vi "Rtde.vi"() -> ()   [LabVIEW 2019]
uses:
  C:/Users/fg/Documents/UniversalRobots.vi/LabVIEW_2024/UnderAutomation.UniversalRobots/lib/UnderAutomation.UniversalRobots.dll
  LabVIEW_2024/UnderAutomation.UniversalRobots/lib/UnderAutomation.UniversalRobots.dll
panel:
  out "Int11":i32
  out "StandardAnalogInput0":dbl
  out "Waveform Z":dbl(graph)
  in  "stop":bool
  in  "Speed":dbl(slide) scale=0.0..1.0
  out "Connected":bool
  out "Error logs":string
  out "Connect error":errorcluster
  # "RTDE with LabVIEW"
  # "Use stop button to properly stop RTDE"
  # "SEND INPUT VALUES"
  # "OUTPUT VALUES EXAMPLE : TCP X at 500HZ"
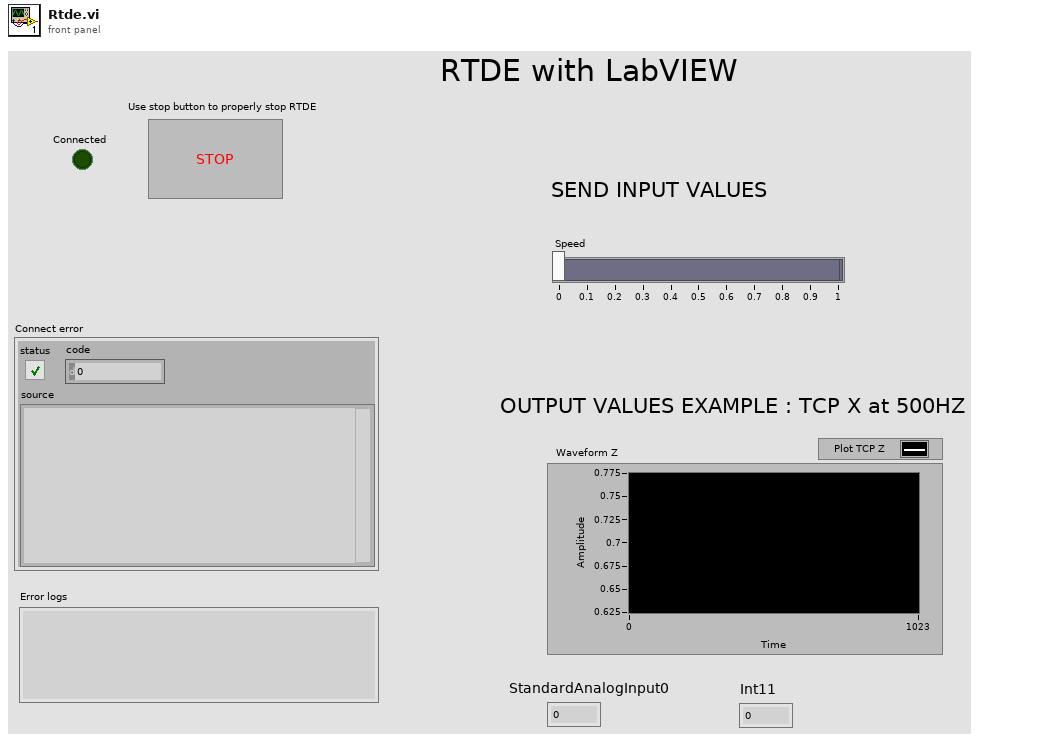
[diagram p1: front panel]
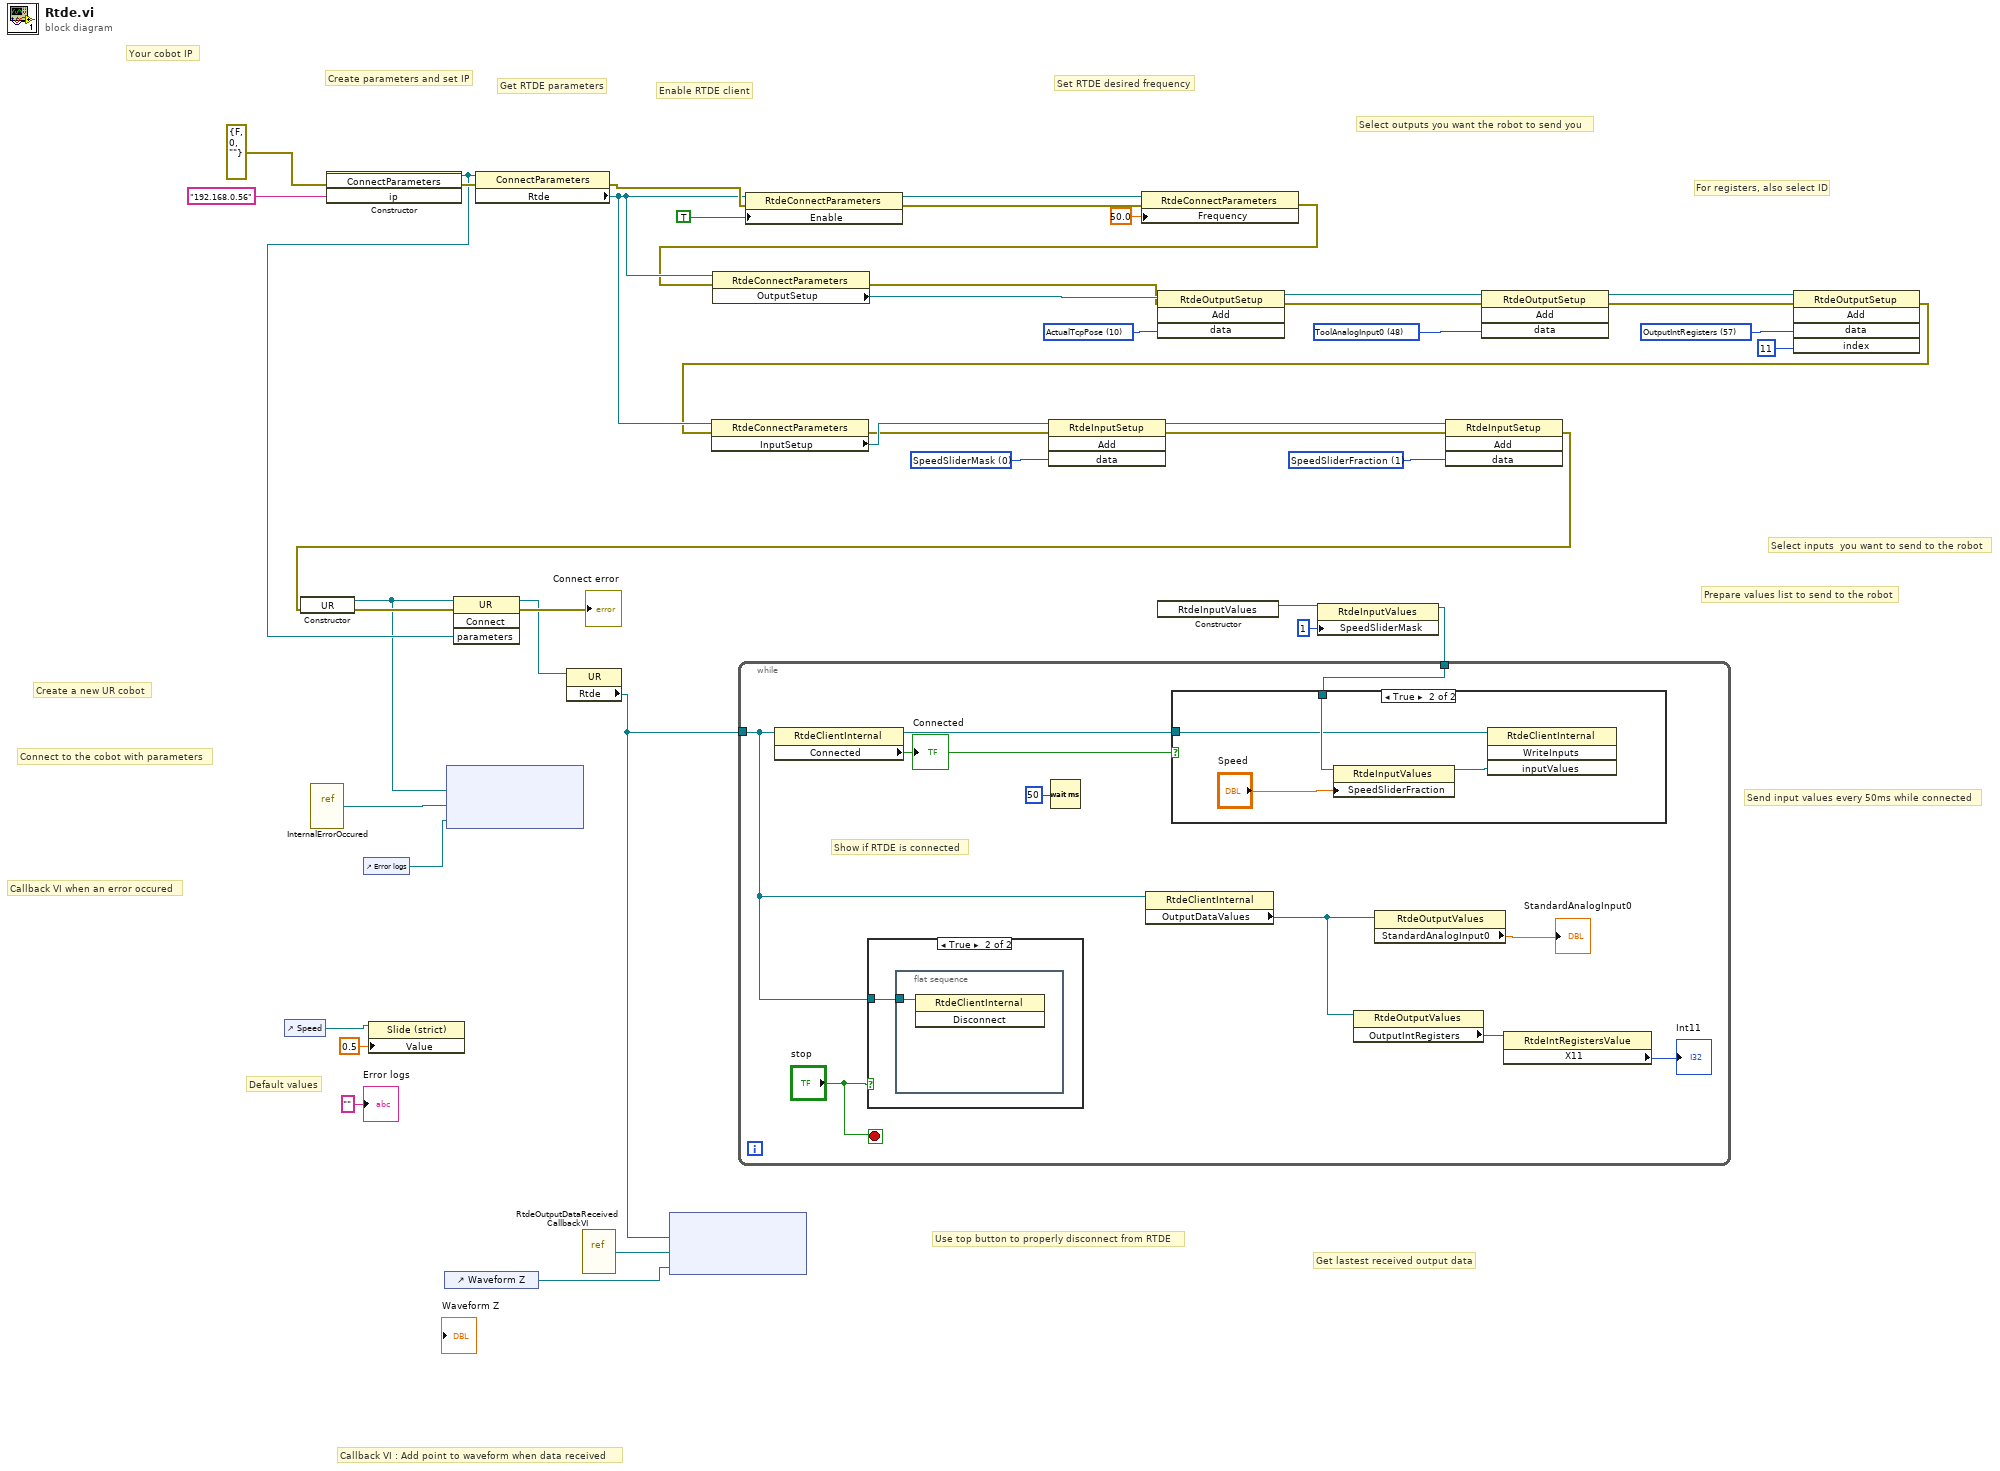
[diagram p0: block diagram]
diagram:
  w26 = 1 items=["SpeedSliderMask", "SpeedSliderFraction", "StandardDigitalOutputMask", "ConfigurableDigitalOutputMask", "StandardDigitalOutput", "ConfigurableDigitalOutput", "StandardAnalogOutputMask", "StandardAnalogOutputType", "StandardAnalogOutput0", "StandardAnalogOutput1", "InputBtRegisters0To31", "InputBtRegisters32To63", "InputBitRegisters", "InputIntRegisters", "InputDoubleRegisters", "ExternalForceTorque"] ("data")
  w28 = 0 items=["SpeedSliderMask", "SpeedSliderFraction", "StandardDigitalOutputMask", "ConfigurableDigitalOutputMask", "StandardDigitalOutput", "ConfigurableDigitalOutput", "StandardAnalogOutputMask", "StandardAnalogOutputType", "StandardAnalogOutput0", "StandardAnalogOutput1", "InputBtRegisters0To31", "InputBtRegisters32To63", "InputBitRegisters", "InputIntRegisters", "InputDoubleRegisters", "ExternalForceTorque"] ("data")
  w38 = 57 items=["Timestamp", "TargetQ", "TargetQd", "TargetQdd", "TargetCurrent", "TargetMoment", "ActualQ", "ActualQd", "ActualCurrent", "JointControlOutput", "ActualTcpPose", "ActualTcpSpeed", "ActualTcpForce", "TargetTcpPose", "TargetTcpSpeed", "ActualDigitalInputBits", "JointTemperatures", "ActualExecutionTime", "RobotMode", "JointMode", "SafetyMode", "SafetyStatus", "ActualToolAccelerometer", "SpeedScaling", "TargetSpeedFraction", "ActualMomentum", "ActualMainVoltage", "ActualRobotVoltage", "ActualRobotCurrent", "ActualJointVoltage", "ActualDigitalOutputBits", "RuntimeState", "ElbowPosition", "ElbowVelocity", "RobotStatusBits", "SafetyStatusBits", "AnalogIOTypes", "StandardAnalogInput0", "StandardAnalogInput1", "StandardAnalogOutput0", "StandardAnalogOutput1", "IOCurrent", "Euromap67InputBits", "Euromap67OutputBits", "Euromap67_24VVoltage", "Euromap67_24VCurrent", "ToolMode", "ToolAnalogInputTypes", "ToolAnalogInput0", "ToolAnalogInput1", "ToolOutputVoltage", "ToolOutputCurrent", "ToolTemperature", "TcpForceScalar", "OutputBitRegisters0To31", "OutputBitRegisters32To63", "OutputBitRegisters", "OutputIntRegisters", "OutputDoubleRegisters", "InputBitRegisters0To31", "InputBitRegisters32To63", "InputBitRegisters", "InputIntRegisters", "InputDoubleRegisters", "ToolOutputMode", "ToolDigitalOutput0mode", "ToolDigitalOutput1Mode", "Payload", "PayloadCOG", "PayloadInertia", "ScriptControlLine", "FTRawWrench"] ("data")
  w40 = 48 items=["Timestamp", "TargetQ", "TargetQd", "TargetQdd", "TargetCurrent", "TargetMoment", "ActualQ", "ActualQd", "ActualCurrent", "JointControlOutput", "ActualTcpPose", "ActualTcpSpeed", "ActualTcpForce", "TargetTcpPose", "TargetTcpSpeed", "ActualDigitalInputBits", "JointTemperatures", "ActualExecutionTime", "RobotMode", "JointMode", "SafetyMode", "SafetyStatus", "ActualToolAccelerometer", "SpeedScaling", "TargetSpeedFraction", "ActualMomentum", "ActualMainVoltage", "ActualRobotVoltage", "ActualRobotCurrent", "ActualJointVoltage", "ActualDigitalOutputBits", "RuntimeState", "ElbowPosition", "ElbowVelocity", "RobotStatusBits", "SafetyStatusBits", "AnalogIOTypes", "StandardAnalogInput0", "StandardAnalogInput1", "StandardAnalogOutput0", "StandardAnalogOutput1", "IOCurrent", "Euromap67InputBits", "Euromap67OutputBits", "Euromap67_24VVoltage", "Euromap67_24VCurrent", "ToolMode", "ToolAnalogInputTypes", "ToolAnalogInput0", "ToolAnalogInput1", "ToolOutputVoltage", "ToolOutputCurrent", "ToolTemperature", "TcpForceScalar", "OutputBitRegisters0To31", "OutputBitRegisters32To63", "OutputBitRegisters", "OutputIntRegisters", "OutputDoubleRegisters", "InputBitRegisters0To31", "InputBitRegisters32To63", "InputBitRegisters", "InputIntRegisters", "InputDoubleRegisters", "ToolOutputMode", "ToolDigitalOutput0mode", "ToolDigitalOutput1Mode", "Payload", "PayloadCOG", "PayloadInertia", "ScriptControlLine", "FTRawWrench"] ("data")
  w42 = 10 items=["Timestamp", "TargetQ", "TargetQd", "TargetQdd", "TargetCurrent", "TargetMoment", "ActualQ", "ActualQd", "ActualCurrent", "JointControlOutput", "ActualTcpPose", "ActualTcpSpeed", "ActualTcpForce", "TargetTcpPose", "TargetTcpSpeed", "ActualDigitalInputBits", "JointTemperatures", "ActualExecutionTime", "RobotMode", "JointMode", "SafetyMode", "SafetyStatus", "ActualToolAccelerometer", "SpeedScaling", "TargetSpeedFraction", "ActualMomentum", "ActualMainVoltage", "ActualRobotVoltage", "ActualRobotCurrent", "ActualJointVoltage", "ActualDigitalOutputBits", "RuntimeState", "ElbowPosition", "ElbowVelocity", "RobotStatusBits", "SafetyStatusBits", "AnalogIOTypes", "StandardAnalogInput0", "StandardAnalogInput1", "StandardAnalogOutput0", "StandardAnalogOutput1", "IOCurrent", "Euromap67InputBits", "Euromap67OutputBits", "Euromap67_24VVoltage", "Euromap67_24VCurrent", "ToolMode", "ToolAnalogInputTypes", "ToolAnalogInput0", "ToolAnalogInput1", "ToolOutputVoltage", "ToolOutputCurrent", "ToolTemperature", "TcpForceScalar", "OutputBitRegisters0To31", "OutputBitRegisters32To63", "OutputBitRegisters", "OutputIntRegisters", "OutputDoubleRegisters", "InputBitRegisters0To31", "InputBitRegisters32To63", "InputBitRegisters", "InputIntRegisters", "InputDoubleRegisters", "ToolOutputMode", "ToolDigitalOutput0mode", "ToolDigitalOutput1Mode", "Payload", "PayloadCOG", "PayloadInertia", "ScriptControlLine", "FTRawWrench"] ("data")
  # "Use top button to properly disconnect from RTDE"
  # "Get lastest received output data"
  # "Send input values every 50ms while connected"
  # "Prepare values list to send to the robot"
  # "Callback VI : Add point to waveform when data received"
  # "Default values"
  # "Callback VI when an error occured"
  # "Connect to the cobot with parameters"
  # "Create a new UR cobot"
  # "Your cobot IP"
  # "Create parameters and set IP"
  # "Get RTDE parameters"
  # "Enable RTDE client"
  # "Set RTDE desired frequency"
  # "Select inputs  you want to send to the robot"
  # "For registers, also select ID"
  # "Select outputs you want the robot to send you"
  n1 = control-ref of="Speed"() -> (w2:refnum<vi>)
  n2 = vi-ref "InternalErrorOccured.vi"() -> ("vi reference"=w11:refnum<vi>)
  n3 = constructor class="ConnectParameters"(error in=errorcluster {"status"=FALSE, "code"=0, "source"=""} ("error in (no error)"), "ip"="192.168.0.56") -> (reference out=w16:refnum<k24>, error out=w35:errorcluster)  [unwired: 2 in, 2 out]
  n4 = control-ref of="Error logs"() -> (w12:refnum<vi>)
  n5 = property class="Slide (strict)"(reference=w2, "Value"=0.5) -> ()  [unwired: 1 in, 2 out]
  n6 = control-ref of="Waveform Z"() -> (w4:refnum<vi>)
  n7 = property class="ConnectParameters"(reference=w16, error in=w35) -> (error out=w34:errorcluster, "Rtde"=w30:refnum<k24>)  [unwired: 1 out]
  n8 = vi-ref "RtdeOutputDataReceivedCallbackVI.vi"() -> ("vi reference"=w3:refnum<vi>)
  n9 = property class="RtdeConnectParameters"(reference=w30, error in=w34, "Enable"=TRUE) -> (reference out=w22:refnum<k24>, error out=w20:errorcluster)
  n10 = property class="RtdeConnectParameters"(reference=w22, error in=w20, "Frequency"=50.0) -> (error out=w19:errorcluster)  [unwired: 1 out]
  n11 = property class="RtdeConnectParameters"(reference=w30, error in=w19) -> (error out=w33:errorcluster, "OutputSetup"=w43:refnum<k24>)  [unwired: 1 out]
  n12 = invoke class="RtdeOutputSetup" method="Add"(reference=w43, error in=w33, "data"=w42) -> (reference out=w41:refnum<k24>, error out=w32:errorcluster)  [unwired: 1 in, 2 out]
  n13 = constructor class="RtdeInputValues"() -> (reference out=w9:refnum<k24>)  [unwired: 3 in, 2 out]
  n14 = property class="RtdeInputValues"(reference=w9, "SpeedSliderMask"=u32 1) -> (reference out=w7:refnum<k24>)  [unwired: 1 in, 1 out]
  n15 = invoke class="RtdeOutputSetup" method="Add"(reference=w41, error in=w32, "data"=w40) -> (reference out=w39:refnum<k24>, error out=w31:errorcluster)  [unwired: 1 in, 2 out]
  n16 = invoke class="RtdeOutputSetup" method="Add"(reference=w39, error in=w31, "data"=w38, "index"=11) -> (error out=w25:errorcluster)  [unwired: 1 in, 4 out]
  n17 = property class="RtdeConnectParameters"(reference=w30, error in=w25) -> (error out=w24:errorcluster, "InputSetup"=w29:refnum<k24>)  [unwired: 1 out]
  n18 = invoke class="RtdeInputSetup" method="Add"(reference=w29, error in=w24, "data"=w28) -> (reference out=w27:refnum<k24>, error out=w23:errorcluster)  [unwired: 1 in, 2 out]
  n19 = invoke class="RtdeInputSetup" method="Add"(reference=w27, error in=w23, "data"=w26) -> (error out=w17:errorcluster)  [unwired: 1 in, 3 out]
  n20 = constructor class="UR"(error in=w17) -> (reference out=w6:refnum<k24>, error out=w18:errorcluster)  [unwired: 2 in, 1 out]
  n21 = node(w6, w11, w12) -> ()  [unwired: 2 in, 2 out]
  n22 = invoke class="UR" method="Connect"(reference=w6, error in=w18, "parameters"=w16) -> (reference out=w13:refnum<k24>, error out=→"Connect error":errorcluster)  [unwired: 1 in, 2 out]
  n23 = property class="UR"(reference=w13) -> ("Rtde"=w5:refnum<k24>)  [unwired: 1 in, 2 out]
  n24 = node(w5, w3, w4) -> ()  [unwired: 2 in, 2 out]
  n25 = while {
    tunnel: w5 -> [w49]
    tunnel: w7 -> [w52]
    stop <- "stop" stop-if-true
    # "Show if RTDE is connected"
    n26 = property class="RtdeClientInternal"(reference=w49) -> (reference out=w51:refnum<k24>, "Connected"=w53:bool)  [unwired: 1 in, 1 out]
    "Connected" <- w53
    n27 = case shown="True" "stop" {
      tunnel: w49 -> [_ w55]
      frame False {
      }
      frame True {
        n28 = flat-sequence {
          tunnel: w55 -> [w56]
          frame #0 {
            n29 = invoke class="RtdeClientInternal" method="Disconnect"(reference=w56) -> ()  [unwired: 2 in, 3 out]
          }
        }
      }
    }
    n30 = Wait (ms)(milliseconds to wait=u32 50) -> ()  [unwired: 1 out]
    n31 = property class="RtdeClientInternal"(reference=w49) -> ("OutputDataValues"=w47:refnum<k24>)  [unwired: 1 in, 2 out]
    n32 = case shown="True" w53 {
      tunnel: w52 -> [_ w60]
      tunnel: w51 -> [_ w58]
      frame False {
      }
      frame True {
        n33 = property class="RtdeInputValues"(reference=w60, "SpeedSliderFraction"="Speed") -> (reference out=w57:refnum<k24>)  [unwired: 1 in, 1 out]
        n34 = invoke class="RtdeClientInternal" method="WriteInputs"(reference=w58, "inputValues"=w57) -> ()  [unwired: 2 in, 4 out]
      }
    }
    n35 = property class="RtdeOutputValues"(reference=w47) -> ("OutputIntRegisters"=w46:refnum<k24>)  [unwired: 1 in, 2 out]
    n36 = property class="RtdeOutputValues"(reference=w47) -> ("StandardAnalogInput0"=→"StandardAnalogInput0":dbl)  [unwired: 1 in, 2 out]
    n37 = property class="RtdeIntRegistersValue"(reference=w46) -> ("X11"=→"Int11":i32)  [unwired: 1 in, 2 out]
  }
  "Error logs" <- "" ("Error logs")
